vi "ESC_StdSci_WorkBench_fnl.vi"() -> ()   [LabVIEW 2015]
uses:
  ESC_StdSci_Driver/SCI_DataPck.ctl
  ESC_StdSci_Driver/SCI_DataType.ctl
panel:
  out "转速_Fault（rpm）":dbl
  out "FeedBack_PWM_NUM_Predicted":i16
  out "FeedBack_PWM_NUM_Measured":i16
  out "霍尔观察器状态机":string
  out "State_HallObStateMachine":u16 format="%x"
  out "测试":waveform(dbl)[](graph) caption="伺服代码效率"
  out "status_TX_overrun":bool
  out "FeedBack_ReferenceError":i32 format="%x"
  out "FeedBack_SpeedReference":i32 format="%x"
  out "FeedBack_ReferenceError_H16":u16 format="%x"
  out "FeedBack_ReferenceError_L16":u16 format="%x"
  out "FeedBack_SpeedReference_H16":u16 format="%x"
  out "status_startup_fail":bool
  out "status_pwm_duty_loop":bool
  out "status_open_loop":bool
  out "status_hall_error":bool
  out "status_open_phase":bool
  out "status_Vbus_undervoltage":bool
  out "status_Vbus_overvoltage":bool
  out "status_motor_stall":bool
  out "status_lose_angle":bool
  out "status_closed_loop":bool
  out "status_over_current":bool
  out "status_motor_enabled":bool
  out "转速（rpm）":dbl
  out "电流":waveform(dbl)[](graph) caption="伺服代码效率"
  out "x/y 2":dbl
  out "TEST3:TEST2":u32 format="%x"
  out "FeedBack_Test3":u16 format="%x"
  out "FeedBack_SpeedAverage":i32 format="%x"
  out "代码效率":waveform(dbl)[](graph) caption="伺服代码效率"
  out "FeedBack_Test0":u16 format="%x"
  out "FeedBack_Test1":u16 format="%x"
  out "FeedBack_Test2":u16 format="%x"
  out "FeedBack_CDE_SMC":u16 format="%x"
  out "FeedBack_CDE_SMM":u16 format="%x"
  out "FeedBack_HallState":u16
  in  "目标转速":u16
  in  "发送_0x02":bool
  in  "输入数据包 4th":T1={"包头"=170, "数据低8位"=0, "数据低高8位"=0, "数据类型"=0, "CRC余数"=0, "数据无效"=FALSE, "数据更新"=FALSE} {"包头" format="%02x"; "数据低8位" format="%02x"; "数据低高8位" format="%02x"; "数据类型" items=["VOID"]; "CRC余数" format="%02x"}
  out "目标转速反馈":u16
  out "串口预写入数据":T1={"包头"=170, "数据低8位"=0, "数据低高8位"=0, "数据类型"=0, "CRC余数"=0, "数据无效"=FALSE, "数据更新"=FALSE} {"包头" format="%02x"; "数据低8位" format="%02x"; "数据低高8位" format="%02x"; "数据类型" items=["VOID"]; "CRC余数" format="%02x"}
  out "控制状态机状态":string
  out "目标占空比反馈":u16
  in  "目标占空比":u16
  in  "发送_0x03":bool
  in  "输入数据包 3rd":T1={"包头"=170, "数据低8位"=0, "数据低高8位"=0, "数据类型"=0, "CRC余数"=0, "数据无效"=FALSE, "数据更新"=FALSE} {"包头" format="%02x"; "数据低8位" format="%02x"; "数据低高8位" format="%02x"; "数据类型" items=["VOID"]; "CRC余数" format="%02x"}
  out "停止":bool=TRUE
  out "起动":bool=TRUE
  out "电机控制指令反馈":u16 format="%x"
  out "主状态机状态":string
  in  "输入数据包 2nd":T1={"包头"=170, "数据低8位"=0, "数据低高8位"=0, "数据类型"=0, "CRC余数"=0, "数据无效"=FALSE, "数据更新"=FALSE} {"包头" format="%02x"; "数据低8位" format="%02x"; "数据低高8位" format="%02x"; "数据类型" items=["VOID"]; "CRC余数" format="%02x"}
  in  "发送_0x01":bool
  in  "输入数据包 1st":T1={"包头"=170, "数据低8位"=0, "数据低高8位"=0, "数据类型"=0, "CRC余数"=0, "数据无效"=FALSE, "数据更新"=FALSE} {"包头" format="%02x"; "数据低8位" format="%02x"; "数据低高8位" format="%02x"; "数据类型" items=["VOID"]; "CRC余数" format="%02x"}
  in  "电机控制指令":u16 format="%x"
  out "转速":waveform(dbl)[](graph) caption="伺服代码效率"
  out "FeedBack_SpeedAverage_L16":u16 format="%x"
  out "FeedBack_SpeedAverage_H16":u16 format="%x"
  out "FeedBack_SpeedReference_L16":u16 format="%x"
  out "FeedBack_AppStatus":u16 format="%x"
  out "FeedBack_iBus":u16 format="%x"
  out "FeedBack_PwmDuty":u16 format="%x"
  out "State_MainStateMachine":u16 format="%x"
  out "State_ControlStateMachine":u16 format="%x"
  out "Config_SpeedPid_Ki":u16 format="%x"
  out "Config_SpeedPid_Kp":u16 format="%x"
  out "CMD_TargetCurrent":u16 format="%x"
  out "CMD_TargetDuty":u16 format="%x"
  out "CMD_TargetSpeed":u16 format="%x"
  out "CMD_MotorEnable":u16 format="%x"
  out "串口读缓存字符数":u32
  in  "VISA资源名称":refnum<visa-resource-name>="COM1"
  out "串口读数据":i32[](array[numeric]) format="%04x"
  out "串口缓存非空":bool
  out "串口写入数据":string
  out "串口读数据包":T1={"包头"=170, "数据低8位"=0, "数据低高8位"=0, "数据类型"=0, "CRC余数"=0, "数据无效"=FALSE, "数据更新"=FALSE} {"包头" format="%02x"; "数据低8位" format="%02x"; "数据低高8位" format="%02x"; "数据类型" items=["VOID"]; "CRC余数" format="%02x"}
  out "串口预写入簇":T1={"包头"=170, "数据低8位"=0, "数据低高8位"=0, "数据类型"=0, "CRC余数"=0, "数据无效"=FALSE, "数据更新"=FALSE} {"包头" format="%02x"; "数据低8位" format="%02x"; "数据低高8位" format="%02x"; "数据类型" items=["VOID"]; "CRC余数" format="%02x"}
  out "写数据更新":bool
  in  "串口写数据包":T1={"包头"=170, "数据低8位"=0, "数据低高8位"=0, "数据类型"=0, "CRC余数"=0, "数据无效"=FALSE, "数据更新"=FALSE} {"包头" format="%02x"; "数据低8位" format="%02x"; "数据低高8位" format="%02x"; "数据类型" items=["VOID"]; "CRC余数" format="%02x"}
  in  "写入数据 2":u16 format="%x"
  in  "写入数据类型 2":u16 format="%x"
  in  "发送 2":bool
  out "写数据CRC余数 2":u16 format="%x"
  in  "停止按钮":bool
  in  "读出数据类型":u16=16 format="%02x"
  out "读数据CRC余数":u16 format="%x"
  out "读出数据":u16 format="%x"
  out "包头":u16 format="%x"
  in  "写入数据 1":u16 format="%x"
  in  "写入数据类型 1":u16 format="%x"
  in  "发送 1":bool
  out "写数据CRC余数 1":u16 format="%x"
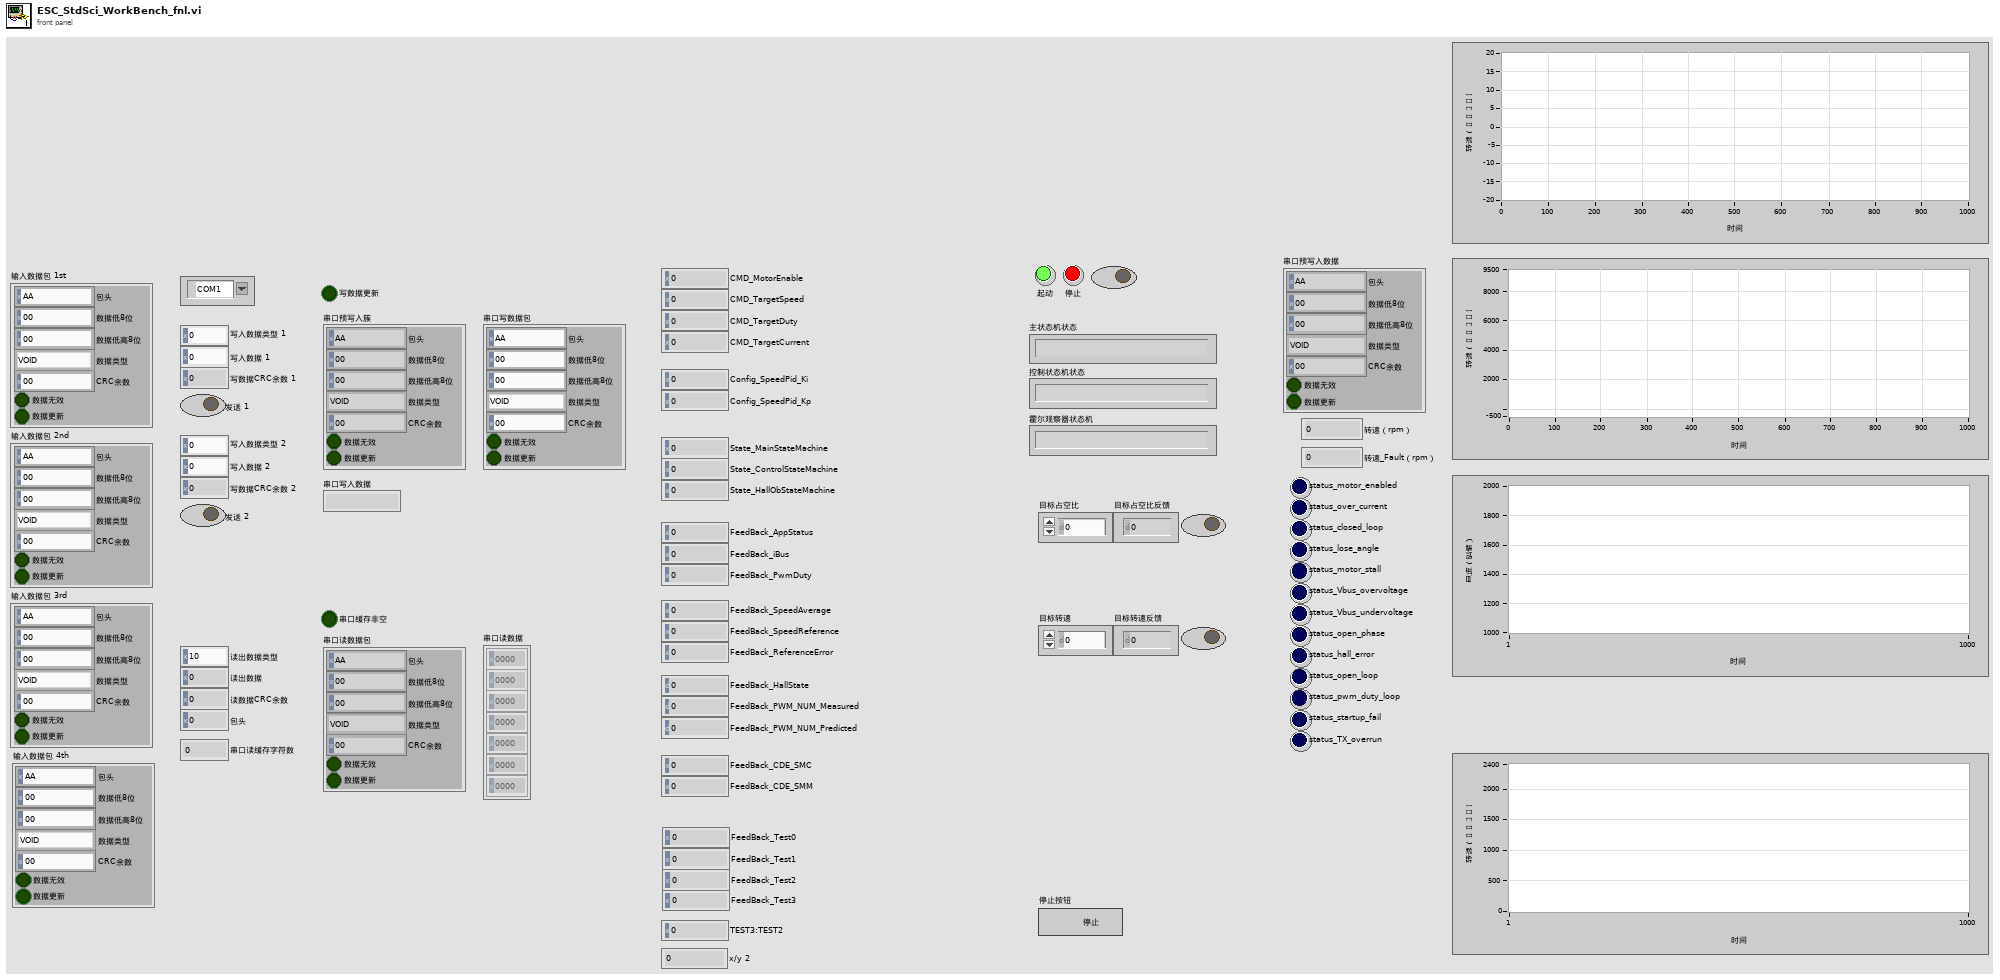
[diagram p1: front panel]
types:
  T1 = typedef "SCI_DataPck.ctl" = cluster{"包头":u16, "数据低8位":u16, "数据低高8位":u16, "数据类型":T2, "CRC余数":u16, "数据无效":bool, "数据更新":bool}
  T2 = typedef "SCI_DataType.ctl" = u16
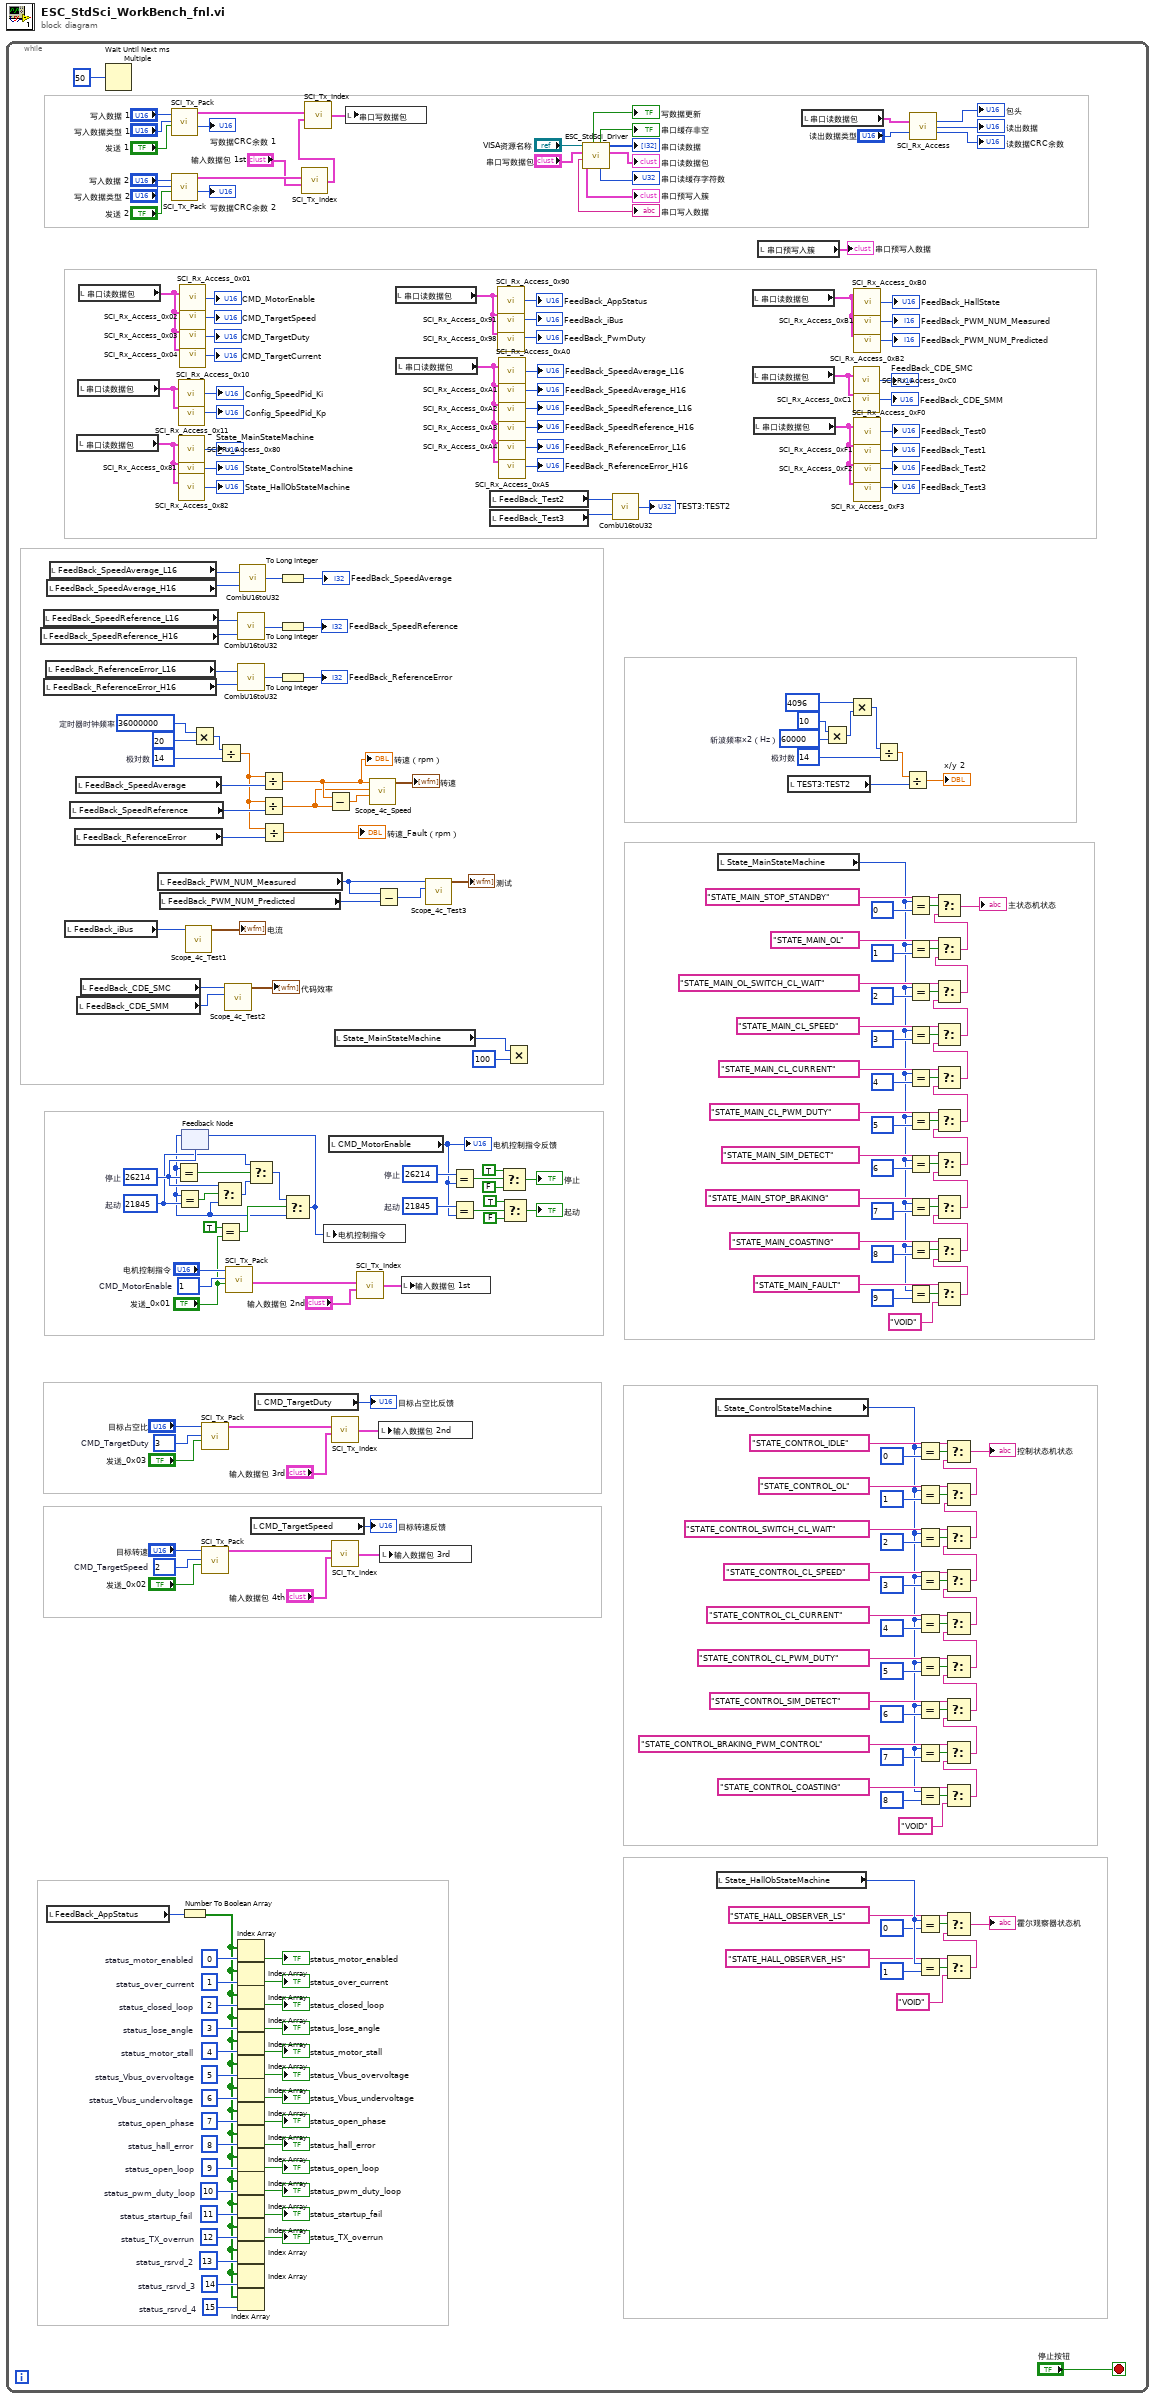
[diagram p0: block diagram]
diagram:
  n1 = while {
    stop <- "停止按钮" stop-if-true
    w63 = u16 15  # status_rsrvd_4
    w62 = u16 14  # status_rsrvd_3
    w64 = u16 13  # status_rsrvd_2
    w65 = u16 12  # status_TX_overrun
    w60 = u16 11  # status_startup_fail
    w61 = u16 10  # status_pwm_duty_loop
    w59 = u16 9  # status_open_loop
    w58 = u16 8  # status_hall_error
    w68 = u16 7  # status_open_phase
    w69 = u16 6  # status_Vbus_undervoltage
    w67 = u16 5  # status_Vbus_overvoltage
    w66 = u16 4  # status_motor_stall
    w71 = u16 3  # status_lose_angle
    w70 = u16 2  # status_closed_loop
    w72 = u16 1  # status_over_current
    w73 = u16 0  # status_motor_enabled
    w85 = u32 14  # 极对数
    w83 = u32 60000  # 斩波频率x2（Hz）
    w108 = u16 2  # CMD_TargetSpeed
    w210 = 36000000  # 定时器时钟频率
    w209 = u32 14  # 极对数
    w218 = u16 3  # CMD_TargetDuty
    w231 = u16 21845  # 起动
    w232 = u16 26214  # 停止
    w233 = u16 21845  # 起动
    w236 = u16 26214  # 停止
    w245 = u16 1  # CMD_MotorEnable
    n2 = local read "FeedBack_SpeedReference_H16"() -> (w39:u16)
    n3 = local read "FeedBack_SpeedReference_L16"() -> (w38:u16)
    n4 = local read "FeedBack_ReferenceError_H16"() -> (w36:u16)
    n5 = local read "FeedBack_ReferenceError_L16"() -> (w37:u16)
    n6 = local read "FeedBack_SpeedAverage_H16"() -> (w96:u16)
    n7 = local read "FeedBack_AppStatus"() -> (w74:u16)
    n8 = local read "FeedBack_SpeedAverage_L16"() -> (w97:u16)
    n9 = local read "FeedBack_iBus"() -> (w44:u16)
    n10 = local read "FeedBack_SpeedReference"() -> (w22:i32)
    n11 = local read "FeedBack_ReferenceError"() -> (w2:i32)
    n12 = local read "FeedBack_SpeedAverage"() -> (w23:i32)
    n13 = local read "串口读数据包"() -> (w21:T1)
    n14 = local read "FeedBack_CDE_SMM"() -> (w76:u16)
    n15 = local read "串口读数据包"() -> (w208:T1)
    n16 = local read "串口读数据包"() -> (w196:T1)
    n17 = local read "FeedBack_CDE_SMC"() -> (w77:u16)
    n18 = Wait Until Next ms Multiple(millisecond multiple=50) -> ()  [unwired: 1 out]
    n19 = local read "FeedBack_PWM_NUM_Measured"() -> (w4:i16)
    n20 = local read "FeedBack_PWM_NUM_Predicted"() -> (w6:i16)
    n21 = call "SCI_Tx_Pack.vi"("数据有效"="发送 1", "数据类型"="写入数据类型 1", "数据"="写入数据 1") -> ("CRC余数"=→"写数据CRC余数 1":u16, "数据包输出"=w252:T1)  [unwired: 7 in]
    n22 = call "SCI_Tx_Pack.vi"("数据有效"="发送 2", "数据类型"="写入数据类型 2", "数据"="写入数据 2") -> ("CRC余数"=→"写数据CRC余数 2":u16, "数据包输出"=w253:T1)  [unwired: 7 in]
    n23 = call "SCI_Rx_Access_0x10.vi"("串口读数据包（簇）"=w208) -> ("数据输出"=→"Config_SpeedPid_Ki":u16)  [unwired: 12 in, 2 out]
    n24 = call "SCI_Rx_Access_0x11.vi"("串口读数据包（簇）"=w208) -> ("数据输出"=→"Config_SpeedPid_Kp":u16)  [unwired: 12 in, 2 out]
    n25 = call "SCI_Rx_Access_0x80.vi"("串口读数据包（簇）"=w21) -> ("数据输出"=→"State_MainStateMachine":u16)  [unwired: 12 in, 2 out]
    n26 = call "SCI_Rx_Access_0x81.vi"("串口读数据包（簇）"=w21) -> ("数据输出"=→"State_ControlStateMachine":u16)  [unwired: 12 in, 2 out]
    n27 = call "SCI_Rx_Access_0x82.vi"("串口读数据包（簇）"=w21) -> ("数据输出"=→"State_HallObStateMachine":u16)  [unwired: 12 in, 2 out]
    n28 = call "SCI_Rx_Access_0x01.vi"("串口读数据包（簇）"=w196) -> ("数据输出"=→"CMD_MotorEnable":u16)  [unwired: 12 in, 2 out]
    n29 = call "SCI_Rx_Access_0x02.vi"("串口读数据包（簇）"=w196) -> ("数据输出"=→"CMD_TargetSpeed":u16)  [unwired: 12 in, 2 out]
    n30 = call "SCI_Rx_Access_0x03.vi"("串口读数据包（簇）"=w196) -> ("数据输出"=→"CMD_TargetDuty":u16)  [unwired: 12 in, 2 out]
    n31 = call "SCI_Rx_Access_0x04.vi"("串口读数据包（簇）"=w196) -> ("数据输出"=→"CMD_TargetCurrent":u16)  [unwired: 12 in, 2 out]
    n32 = feedback #1(w236) -> (w214:u16)
    n33 = Equal?(x=w214, y=w236) -> (x = y?=w241:bool)
    n34 = Equal?(x=w214, y=w233) -> (x = y?=w240:bool)
    n35 = Number To Boolean Array(number=w74) -> (Boolean array=w57:bool[])
    n36 = call "Scope_4c_Test1.vi"("Channel 1"=w44) -> ("Display"=→"电流":waveform(dbl)[])  [unwired: 10 in]
    n37 = Multiply(x=w210, y=20) -> (x*y=w34:i32)
    n38 = call "SCI_Tx_Pack.vi"("数据有效"="发送_0x03", "数据类型"=w218, "数据"="目标占空比") -> ("数据包输出"=w217:T1)  [unwired: 7 in, 1 out]
    n39 = call "SCI_Tx_Pack.vi"("数据有效"="发送_0x02", "数据类型"=w108, "数据"="目标转速") -> ("数据包输出"=w109:T1)  [unwired: 7 in, 1 out]
    n40 = Select(t=w236, s=w240, f=w214) -> (s? t:f=w239:u16)
    n41 = Equal?(x=TRUE, y="发送_0x01") -> (x = y?=w235:bool)
    n42 = Divide(x=w34, y=w209) -> (x/y=w1:dbl)
    n43 = call "Scope_4c_Test2.vi"("Channel 2"=w76, "Channel 1"=w77) -> ("Display"=→"代码效率":waveform(dbl)[])  [unwired: 9 in]
    n44 = call "SCI_Tx_Pack.vi"("数据有效"="发送_0x01", "数据类型"=w245, "数据"="电机控制指令") -> ("数据包输出"=w246:T1)  [unwired: 7 in, 1 out]
    n45 = call "CombU16toU32.vi"("数据高16位"=w39, "数据低16位"=w38) -> ("32位数据输出"=w31:u32)
    n46 = call "CombU16toU32.vi"("数据高16位"=w36, "数据低16位"=w37) -> ("32位数据输出"=w30:u32)
    n47 = Index Array(array=w57, index=w73) -> (element=→"status_motor_enabled":bool)
    n48 = Index Array(array=w57, index=w72) -> (element=→"status_over_current":bool)
    n49 = Index Array(array=w57, index=w70) -> (element=→"status_closed_loop":bool)
    n50 = Index Array(array=w57, index=w71) -> (element=→"status_lose_angle":bool)
    n51 = Index Array(array=w57, index=w66) -> (element=→"status_motor_stall":bool)
    n52 = Index Array(array=w57, index=w67) -> (element=→"status_Vbus_overvoltage":bool)
    n53 = Index Array(array=w57, index=w69) -> (element=→"status_Vbus_undervoltage":bool)
    n54 = Index Array(array=w57, index=w68) -> (element=→"status_open_phase":bool)
    n55 = Index Array(array=w57, index=w58) -> (element=→"status_hall_error":bool)
    n56 = Index Array(array=w57, index=w59) -> (element=→"status_open_loop":bool)
    n57 = Index Array(array=w57, index=w61) -> (element=→"status_pwm_duty_loop":bool)
    n58 = Index Array(array=w57, index=w60) -> (element=→"status_startup_fail":bool)
    n59 = Index Array(array=w57, index=w65) -> (element=→"status_TX_overrun":bool)
    n60 = Index Array(array=w57, index=w64) -> ()  [unwired: 1 out]
    n61 = Index Array(array=w57, index=w62) -> ()  [unwired: 1 out]
    n62 = Index Array(array=w57, index=w63) -> ()  [unwired: 1 out]
    n63 = call "CombU16toU32.vi"("数据高16位"=w96, "数据低16位"=w97) -> ("32位数据输出"=w33:u32)
    n64 = Select(t=w233, s=w241, f=w239) -> (s? t:f=w237:u16)
    n65 = local read "CMD_TargetSpeed"() -> (→"目标转速反馈":u16)
    n66 = local read "CMD_TargetDuty"() -> (→"目标占空比反馈":u16)
    n67 = Divide(x=w1, y=w23) -> (x/y=w26:dbl)
    "转速（rpm）" <- w26
    n68 = Divide(x=w1, y=w22) -> (x/y=w24:dbl)
    n69 = Divide(x=w1, y=w2) -> (x/y=→"转速_Fault（rpm）":dbl)
    n70 = To Long Integer(number=w33) -> (32bit integer=→"FeedBack_SpeedAverage":i32)
    n71 = To Long Integer(number=w31) -> (32bit integer=→"FeedBack_SpeedReference":i32)
    n72 = To Long Integer(number=w30) -> (32bit integer=→"FeedBack_ReferenceError":i32)
    n73 = Select(t=w237, s=w235, f=w214) -> (s? t:f=w213:u16)
    n74 = feedback-in #1(w213) -> ()
    n75 = call "SCI_Tx_Index.vi"("输入数据包（簇）"=w253, "下一包数据（簇）"="输入数据包 1st") -> ("上一个包数据（簇）"=w250:T1)  [unwired: 5 in]
    n76 = call "SCI_Tx_Index.vi"("输入数据包（簇）"=w252, "下一包数据（簇）"=w250) -> ("上一个包数据（簇）"=w251:T1)  [unwired: 5 in]
    n77 = local write "电机控制指令"(w213) -> ()
    n78 = Subtract(x=w26, y=w24) -> (x-y=w25:dbl)
    n79 = local read "CMD_MotorEnable"() -> (w230:u16)
    "电机控制指令反馈" <- w230
    n80 = call "SCI_Tx_Index.vi"("输入数据包（簇）"=w217, "下一包数据（簇）"="输入数据包 3rd") -> ("上一个包数据（簇）"=w216:T1)  [unwired: 5 in]
    n81 = call "SCI_Tx_Index.vi"("输入数据包（簇）"=w109, "下一包数据（簇）"="输入数据包 4th") -> ("上一个包数据（簇）"=w110:T1)  [unwired: 5 in]
    n82 = local read "State_MainStateMachine"() -> (w81:u16)
    n83 = local write "串口写数据包"(w251) -> ()
    n84 = call "SCI_Tx_Index.vi"("输入数据包（簇）"=w246, "下一包数据（簇）"="输入数据包 2nd") -> ("上一个包数据（簇）"=w244:T1)  [unwired: 5 in]
    n85 = call "Scope_4c_Speed.vi"("Channel 3"=w25, "Channel 2"=w24, "Channel 1"=w26) -> ("Display"=→"转速":waveform(dbl)[])  [unwired: 8 in]
    n86 = Subtract(x=w4, y=w6) -> (x-y=w5:i16)
    n87 = local write "输入数据包 2nd"(w216) -> ()
    n88 = local write "输入数据包 3rd"(w110) -> ()
    n89 = local read "串口读数据包"() -> (w203:T1)
    n90 = local read "串口读数据包"() -> (w43:T1)
    n91 = local write "输入数据包 1st"(w244) -> ()
    n92 = call "Scope_4c_Test3.vi"("Channel 2"=w5, "Channel 1"=w4) -> ("Display"=→"测试":waveform(dbl)[])  [unwired: 9 in]
    n93 = Equal?(x=w232, y=w230) -> (x = y?=w229:bool)
    n94 = Equal?(x=w231, y=w230) -> (x = y?=w223:bool)
    n95 = local read "FeedBack_Test2"() -> (w93:u16)
    n96 = local read "FeedBack_Test3"() -> (w92:u16)
    n97 = call "SCI_Rx_Access_0x90.vi"("串口读数据包（簇）"=w203) -> ("数据输出"=→"FeedBack_AppStatus":u16)  [unwired: 12 in, 2 out]
    n98 = call "SCI_Rx_Access_0x91.vi"("串口读数据包（簇）"=w203) -> ("数据输出"=→"FeedBack_iBus":u16)  [unwired: 12 in, 2 out]
    n99 = call "SCI_Rx_Access_0x98.vi"("串口读数据包（簇）"=w203) -> ("数据输出"=→"FeedBack_PwmDuty":u16)  [unwired: 12 in, 2 out]
    n100 = call "SCI_Rx_Access_0xA0.vi"("串口读数据包（簇）"=w43) -> ("数据输出"=→"FeedBack_SpeedAverage_L16":u16)  [unwired: 12 in, 2 out]
    n101 = call "SCI_Rx_Access_0xA1.vi"("串口读数据包（簇）"=w43) -> ("数据输出"=→"FeedBack_SpeedAverage_H16":u16)  [unwired: 12 in, 2 out]
    n102 = call "SCI_Rx_Access_0xA2.vi"("串口读数据包（簇）"=w43) -> ("数据输出"=→"FeedBack_SpeedReference_L16":u16)  [unwired: 12 in, 2 out]
    n103 = call "SCI_Rx_Access_0xA3.vi"("串口读数据包（簇）"=w43) -> ("数据输出"=→"FeedBack_SpeedReference_H16":u16)  [unwired: 12 in, 2 out]
    n104 = call "SCI_Rx_Access_0xA4.vi"("串口读数据包（簇）"=w43) -> ("数据输出"=→"FeedBack_ReferenceError_L16":u16)  [unwired: 12 in, 2 out]
    n105 = call "SCI_Rx_Access_0xA5.vi"("串口读数据包（簇）"=w43) -> ("数据输出"=→"FeedBack_ReferenceError_H16":u16)  [unwired: 12 in, 2 out]
    n106 = Select(t=TRUE, s=w229, f=FALSE) -> (s? t:f=→"停止":bool)
    n107 = Select(t=TRUE, s=w223, f=FALSE) -> (s? t:f=→"起动":bool)
    n108 = Multiply(x=w81, y=u16 100) -> ()  [unwired: 1 out]
    n109 = call "ESC_StdSci_Driver.vi"("串口写数据包"="串口写数据包", "VISA资源名称"="VISA资源名称") -> ("串口读数据包"=→"串口读数据包":T1, "串口读数据"=→"串口读数据":i32[], "串口读缓存字符数"=→"串口读缓存字符数":u32, "串口缓存非空"=→"串口缓存非空":bool, "写数据更新"=→"写数据更新":bool, "串口写入数据包"=→"串口预写入簇":T1, "串口写入数据"=→"串口写入数据":string)  [unwired: 3 in]
    n110 = call "CombU16toU32.vi"("数据高16位"=w92, "数据低16位"=w93) -> ("32位数据输出"=→"TEST3:TEST2":u32)
    n111 = local read "State_ControlStateMachine"() -> (w113:u16)
    n112 = local read "State_HallObStateMachine"() -> (w19:u16)
    n113 = local read "State_MainStateMachine"() -> (w150:u16)
    n114 = local read "串口读数据包"() -> (w7:T1)
    n115 = local read "串口读数据包"() -> (w103:T1)
    n116 = local read "串口读数据包"() -> (w94:T1)
    n117 = local read "串口预写入簇"() -> (→"串口预写入数据":T1)
    n118 = local read "TEST3:TEST2"() -> (w90:u32)
    n119 = local read "串口读数据包"() -> (w263:T1)
    n120 = Multiply(x=u32 10, y=w83) -> (x*y=w88:u32)
    n121 = Multiply(x=u32 4096, y=w88) -> (x*y=w87:u32)
    n122 = call "SCI_Rx_Access_0xC0.vi"("串口读数据包（簇）"=w103) -> ("数据输出"=→"FeedBack_CDE_SMC":u16)  [unwired: 12 in, 2 out]
    n123 = call "SCI_Rx_Access_0xC1.vi"("串口读数据包（簇）"=w103) -> ("数据输出"=→"FeedBack_CDE_SMM":u16)  [unwired: 12 in, 2 out]
    n124 = call "SCI_Rx_Access_0xB0.vi"("串口读数据包（簇）"=w7) -> ("数据输出"=→"FeedBack_HallState":u16)  [unwired: 12 in, 2 out]
    n125 = call "SCI_Rx_Access_0xB1.vi"("串口读数据包（簇）"=w7) -> ("数据输出"=→"FeedBack_PWM_NUM_Measured":u16)  [unwired: 12 in, 2 out]
    n126 = call "SCI_Rx_Access_0xB2.vi"("串口读数据包（簇）"=w7) -> ("数据输出"=→"FeedBack_PWM_NUM_Predicted":u16)  [unwired: 12 in, 2 out]
    n127 = call "SCI_Rx_Access_0xF0.vi"("串口读数据包（簇）"=w94) -> ("数据输出"=→"FeedBack_Test0":u16)  [unwired: 12 in, 2 out]
    n128 = call "SCI_Rx_Access_0xF1.vi"("串口读数据包（簇）"=w94) -> ("数据输出"=→"FeedBack_Test1":u16)  [unwired: 12 in, 2 out]
    n129 = call "SCI_Rx_Access_0xF2.vi"("串口读数据包（簇）"=w94) -> ("数据输出"=→"FeedBack_Test2":u16)  [unwired: 12 in, 2 out]
    n130 = call "SCI_Rx_Access_0xF3.vi"("串口读数据包（簇）"=w94) -> ("数据输出"=→"FeedBack_Test3":u16)  [unwired: 12 in, 2 out]
    n131 = Divide(x=w87, y=w85) -> (x/y=w86:dbl)
    n132 = Divide(x=w86, y=w90) -> (x/y=→"x/y 2":dbl)
    n133 = Equal?(x=w150, y=u16 0) -> (x = y?=w191:bool)
    n134 = Equal?(x=w150, y=u16 1) -> (x = y?=w187:bool)
    n135 = Equal?(x=w150, y=u16 2) -> (x = y?=w183:bool)
    n136 = Equal?(x=w150, y=u16 3) -> (x = y?=w181:bool)
    n137 = Equal?(x=w150, y=u16 4) -> (x = y?=w177:bool)
    n138 = Equal?(x=w150, y=u16 5) -> (x = y?=w175:bool)
    n139 = Equal?(x=w150, y=u16 6) -> (x = y?=w171:bool)
    n140 = Equal?(x=w150, y=u16 7) -> (x = y?=w169:bool)
    n141 = Equal?(x=w150, y=u16 8) -> (x = y?=w165:bool)
    n142 = Equal?(x=w150, y=u16 9) -> (x = y?=w163:bool)
    n143 = call "SCI_Rx_Access.vi"("串口读数据包（簇）"=w263, "数据类型"="读出数据类型") -> ("包头"=→"包头":u16, "数据输出"=→"读出数据":u16, "CRC余数"=→"读数据CRC余数":u16)  [unwired: 11 in]
    n144 = Equal?(x=w113, y=u16 0) -> (x = y?=w149:bool)
    n145 = Equal?(x=w113, y=u16 1) -> (x = y?=w145:bool)
    n146 = Equal?(x=w113, y=u16 2) -> (x = y?=w141:bool)
    n147 = Equal?(x=w113, y=u16 3) -> (x = y?=w139:bool)
    n148 = Equal?(x=w113, y=u16 4) -> (x = y?=w135:bool)
    n149 = Equal?(x=w113, y=u16 5) -> (x = y?=w133:bool)
    n150 = Equal?(x=w113, y=u16 6) -> (x = y?=w129:bool)
    n151 = Equal?(x=w113, y=u16 7) -> (x = y?=w127:bool)
    n152 = Equal?(x=w113, y=u16 8) -> (x = y?=w123:bool)
    n153 = Equal?(x=w19, y=u16 0) -> (x = y?=w11:bool)
    n154 = Equal?(x=w19, y=u16 1) -> (x = y?=w15:bool)
    n155 = Select(t="STATE_MAIN_FAULT" ("字符串 2"), s=w163, f="VOID" ("字符串 2")) -> (s? t:f=w153:string)
    n156 = Select(t="STATE_MAIN_COASTING" ("字符串 2"), s=w165, f=w153) -> (s? t:f=w154:string)
    n157 = Select(t="STATE_MAIN_STOP_BRAKING" ("字符串 2"), s=w169, f=w154) -> (s? t:f=w155:string)
    n158 = Select(t="STATE_MAIN_SIM_DETECT" ("字符串 2"), s=w171, f=w155) -> (s? t:f=w156:string)
    n159 = Select(t="STATE_MAIN_CL_PWM_DUTY" ("字符串 2"), s=w175, f=w156) -> (s? t:f=w157:string)
    n160 = Select(t="STATE_MAIN_CL_CURRENT" ("字符串 2"), s=w177, f=w157) -> (s? t:f=w158:string)
    n161 = Select(t="STATE_MAIN_CL_SPEED" ("字符串 2"), s=w181, f=w158) -> (s? t:f=w159:string)
    n162 = Select(t="STATE_MAIN_OL_SWITCH_CL_WAIT" ("字符串 2"), s=w183, f=w159) -> (s? t:f=w160:string)
    n163 = Select(t="STATE_MAIN_OL" ("字符串 2"), s=w187, f=w160) -> (s? t:f=w151:string)
    n164 = Select(t="STATE_MAIN_STOP_STANDBY" ("字符串 2"), s=w191, f=w151) -> (s? t:f=→"主状态机状态":string)
    n165 = Select(t="STATE_CONTROL_COASTING" ("字符串 2"), s=w123, f="VOID" ("字符串 2")) -> (s? t:f=w115:string)
    n166 = Select(t="STATE_CONTROL_BRAKING_PWM_CONTROL" ("字符串 2"), s=w127, f=w115) -> (s? t:f=w116:string)
    n167 = Select(t="STATE_CONTROL_SIM_DETECT" ("字符串 2"), s=w129, f=w116) -> (s? t:f=w117:string)
    n168 = Select(t="STATE_CONTROL_CL_PWM_DUTY" ("字符串 2"), s=w133, f=w117) -> (s? t:f=w118:string)
    n169 = Select(t="STATE_CONTROL_CL_CURRENT" ("字符串 2"), s=w135, f=w118) -> (s? t:f=w119:string)
    n170 = Select(t="STATE_CONTROL_CL_SPEED" ("字符串 2"), s=w139, f=w119) -> (s? t:f=w120:string)
    n171 = Select(t="STATE_CONTROL_SWITCH_CL_WAIT" ("字符串 2"), s=w141, f=w120) -> (s? t:f=w121:string)
    n172 = Select(t="STATE_CONTROL_OL" ("字符串 2"), s=w145, f=w121) -> (s? t:f=w114:string)
    n173 = Select(t="STATE_CONTROL_IDLE" ("字符串 2"), s=w149, f=w114) -> (s? t:f=→"控制状态机状态":string)
    n174 = Select(t="STATE_HALL_OBSERVER_HS" ("字符串 2"), s=w15, f="VOID" ("字符串 2")) -> (s? t:f=w18:string)
    n175 = Select(t="STATE_HALL_OBSERVER_LS" ("字符串 2"), s=w11, f=w18) -> (s? t:f=→"霍尔观察器状态机":string)
  }
